vi "Add Basic Info Values.vi"(8 "error in (no error)":errorcluster, 9 "Build Type String":string, 10 "LVLIB Name":string, 11 "Map in":map{string, string}(c390)) -> (0 "error out":errorcluster, 3 "Map out":map{string, string}(c390))   [LabVIEW 2019, in "NIPKG Packager.lvclass"]
uses:
  NIPKG Packager.lvclass
  NIPKG Naming/NIPKG Naming.lvlib
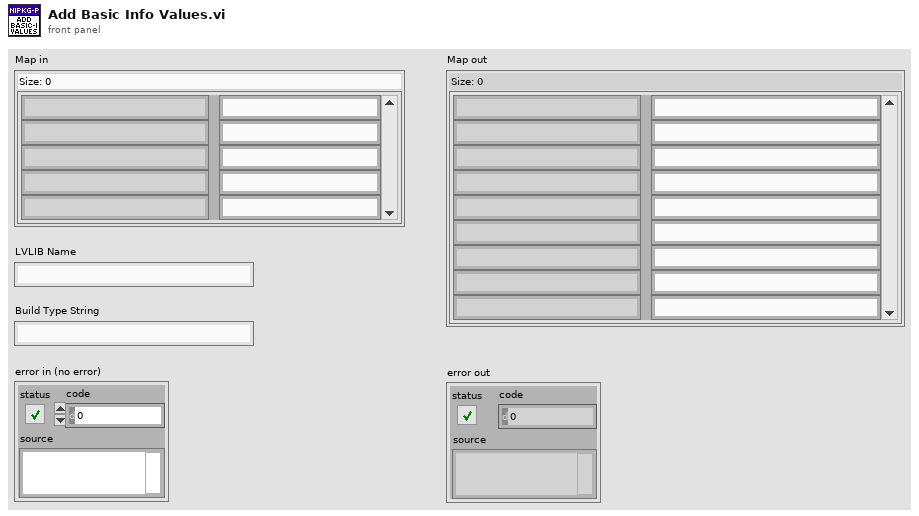
[diagram p1: front panel]
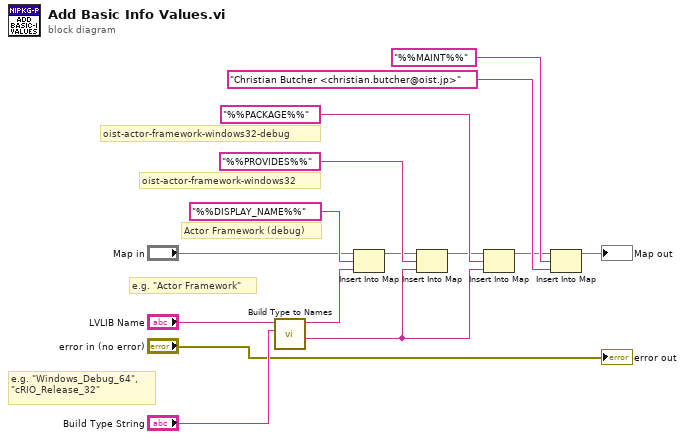
[diagram p0: block diagram]
diagram:
  # "Actor Framework (debug)"
  # "oist-actor-framework-windows32-debug"
  # "oist-actor-framework-windows32"
  # "e.g. \"Windows_Debug_64\", \"cRIO_Release_32\""
  # "e.g. \"Actor Framework\""
  n1 = call "Build Type to Names.vi"("Build Type String"="Build Type String", "Library Name"="LVLIB Name") -> ("Package Name"=w1:string, "Display Name"=w4:string)  [unwired: 6 in, 2 out]
  n2 = Insert Into Map(map in="Map in", key="%%DISPLAY_NAME%%", value=w4) -> (map out=w7:map{string, string})  [unwired: 2 out]
  n3 = Insert Into Map(map in=w7, key="%%PROVIDES%%", value=w1) -> (map out=w6:map{string, string})  [unwired: 2 out]
  n4 = Insert Into Map(map in=w6, key="%%PACKAGE%%", value=w1) -> (map out=w12:map{string, string})  [unwired: 2 out]
  n5 = Insert Into Map(map in=w12, key="%%MAINT%%", value="Christian Butcher <christian.butcher@oist.jp>") -> (map out=→"Map out":map{string, string})  [unwired: 2 out]
  "error out" <- "error in (no error)"
